vi "题目4.vi"() -> ()   [LabVIEW 2017]
panel:
  in  "停止":bool
  in  "枚举":enum16{"张三", "李四", "王五"}(ring)
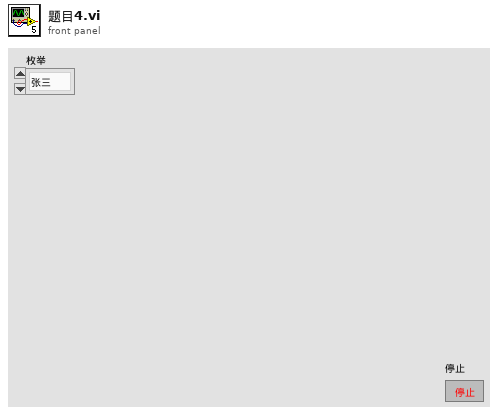
[diagram p1: front panel]
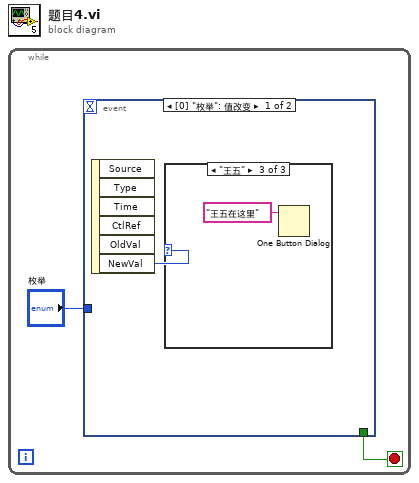
[diagram p0: block diagram]
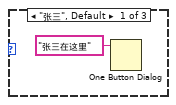
[diagram p2: hidden frame]
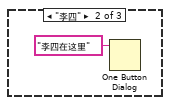
[diagram p3: hidden frame]
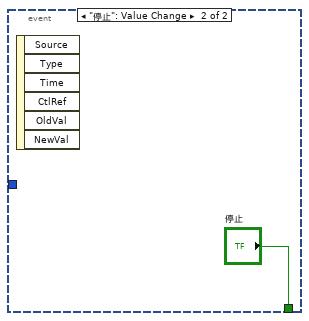
[diagram p4: hidden frame]
diagram:
  n1 = while {
    stop <- w1 stop-if-true
    n2 = event shown="[0] \"枚举\": 值改变" {
      selector: _ -> [_ _]
      dyn-events: _ -> [_ _]
      timeout: _ -> [_ _]
      tunnel: [_ "停止"] -> w1
      tunnel: "枚举" -> [_ _]
      event "枚举": Value Change {
        n3 = event-data() -> ("NewVal"=w3:enum16{"张三", "李四", "王五"})  [unwired: 1 in, 5 out]
        n4 = case shown="\"王五\"" w3 {
          frame "张三", Default {
            n5 = One Button Dialog(message="张三在这里") -> ()  [unwired: 1 in, 1 out]
          }
          frame "李四" {
            n6 = One Button Dialog(message="李四在这里") -> ()  [unwired: 1 in, 1 out]
          }
          frame "王五" {
            n7 = One Button Dialog(message="王五在这里") -> ()  [unwired: 1 in, 1 out]
          }
        }
      }
      event "停止": Value Change {
        n8 = event-data() -> ()  [unwired: 1 in, 6 out]
      }
    }
  }
